vi "EditContact.vi"(7 "LabVIEW Web Service Request":refnum<class "Web Request.lvclass">) -> ()   [LabVIEW 2014]
doc: "This HTTP Method VI accepts a contact as form post data and either updates an existing contact or inserts a new one into the address book data store. It then redirects back to the contact list."
uses:
  <vilib>/wsapi/Web Request.lvclass
  DataManager/StateStore/Controls/DataFunction.ctl
panel:
  # "Because this is an HTTP Method VI, LabVIEW Web Service Request is populated automatically."
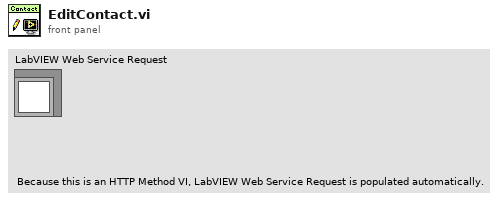
[diagram p1: front panel]
types:
  T1 = typedef "DataFunction.ctl" = enum16{"Initialise", "Release", "Get Data", "Set Data", "Preview Data"}
  T2 = typedef "CData Core Control.ctl" = cluster{"train_data_array":cluster{"uuid":string, "int":i32, "posit_array":cluster{"x":dbl, "y":dbl, "z":dbl}[]}[], "train_control_array":cluster{"uuid":string, "throttle":dbl, "brake":dbl, "horn":dbl, "wait":dbl, "name":string, "mode":string, "dest":string}[], "switch_data_array":cluster{"switch_posit":cluster{"x":dbl, "y":dbl, "z":dbl}, "manual":bool}[], "switch_control_array":cluster{"switch_posit":cluster{"x":dbl, "y":dbl, "z":dbl}, "switch":bool, "invert":bool, "wait":dbl}[]}
  T3 = cluster{"train_data":cluster{"uuid":string, "int":i32, "posit_array":cluster{"x":dbl, "y":dbl, "z":dbl}[]}, "train_control":cluster{"uuid":string, "throttle":dbl, "brake":dbl, "horn":dbl, "wait":dbl, "name":string, "mode":string, "dest":string}}
  T4 = typedef "Contact Data.lvlib/DestinationCluster.ctl" = cluster{"Desination":string, "DestControls":T5, "Timer":u32, "Set Timer":u32, "Time Stamp":timestamp, "Repeat?":bool, "Optional Data":string, "Distance":dbl}
  T5 = typedef "Contact Data.lvlib/DesinationControls.ctl" = enum16{"Tracker", "Manual", "Stop", "Station DateTime", "Station Timer", "Maintain"}
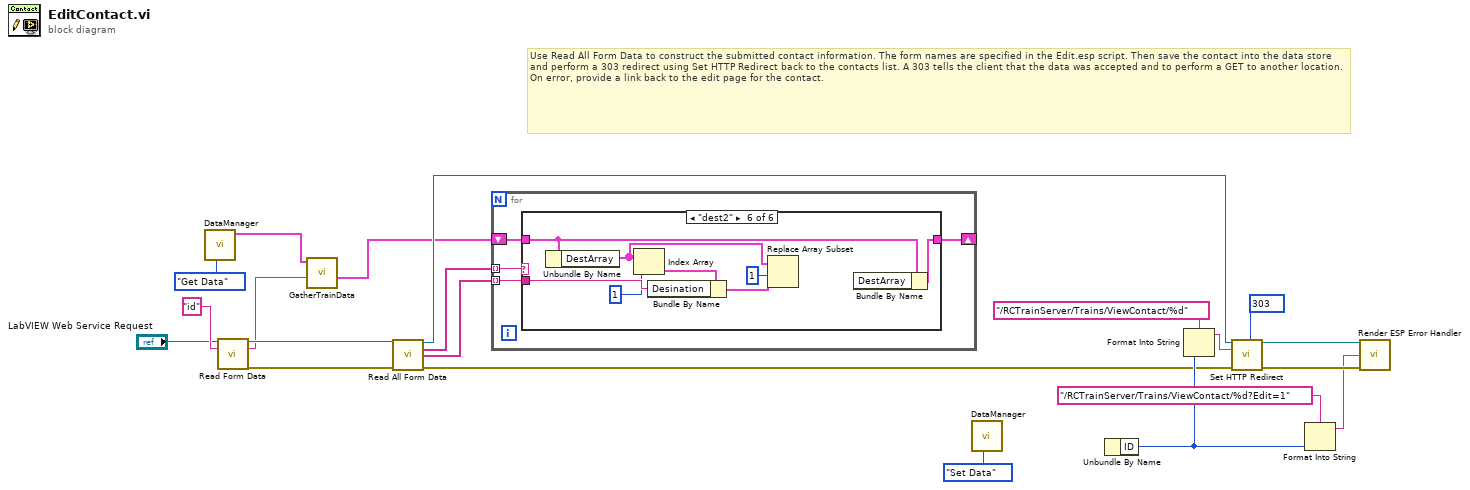
[diagram p0: block diagram]
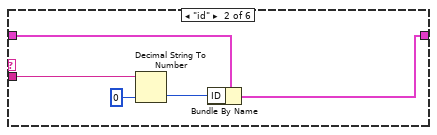
[diagram p3: hidden frame]
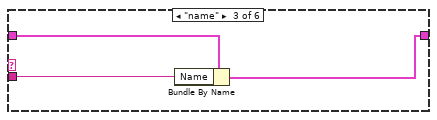
[diagram p4: hidden frame]
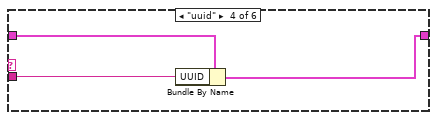
[diagram p5: hidden frame]
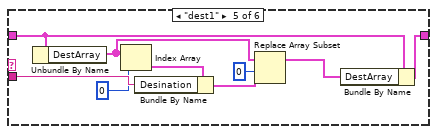
[diagram p6: hidden frame]
diagram:
  w21 = 303 items=["100"=100, "101"=101, "200"=200, "201"=201, "202"=202, "203"=203, "204"=204, "205"=205, "206"=206, "300"=300, "301"=301, "302"=302, "303"=303, "304"=304, "305"=305, "306"=306, "307"=307, "400"=400, "401"=401, "402"=402, "403"=403, "404"=404, "405"=405, "406"=406, "407"=407, "408"=408, "409"=409, "410"=410, "411"=411, "412"=412, "413"=413, "414"=414, "415"=415, "416"=416, "417"=417, "500"=500, "501"=501, "502"=502, "503"=503, "504"=504, "505"=505] ("response code (307)")
  # "Use Read All Form Data to construct the submitted contact information. The form names are specified in the Edit.esp script. Then save the contact into the data store and perform a 303 redirect using Set HTTP Redirect back to the contacts list. A 303 tells the client that the data was accepted and to perform a GET to another location. On error, provide a link back to the edit page for the contact."
  n1 = call "DataManager.vi"("DataFunction"=DataFunction."Get Data") -> ("CData Out"=w5:T2)  [unwired: 9 in, 1 out]
  n2 = call <vilib>:"Read Form Data.vi"("LabVIEW Web Service Request"="LabVIEW Web Service Request", "key"="id") -> ("LabVIEW Web Service Request out"=w11:refnum<class "Web Request.lvclass">, "value"=w6:string, "error out"=w10:errorcluster)  [unwired: 10 in, 1 out]
  n3 = call "GatherTrainData.vi"("uuid"=w6, "CData Out"=w5) -> ("Cluster"=w3:T3)  [unwired: 7 in, 2 out]
  n4 = call <vilib>:"Read All Form Data.vi"("LabVIEW Web Service Request"=w11, "error in (no error)"=w10) -> ("LabVIEW Web Service Request out"=w17:refnum<class "Web Request.lvclass">, "Key"=w19:string[], "Value"=w18:string[], "error out"=w1:errorcluster)  [unwired: 9 in, 1 out]
  n5 = for {
    tunnel: w19 -> [w25] mode=indexing
    tunnel: w18 -> [w24] mode=indexing
    shift-right: [w22] -> _
    shift-left: w3 -> [w23]
    n6 = case shown="\"dest2\"" w25 {
      tunnel: w24 -> [_ w29 w32 w36 w43 w51]
      tunnel: w23 -> [w26 w31 w34 w37 w45 w53]
      tunnel: [w26 w30 w33 w35 w46 w54] -> w22
      frame Default {
      }
      frame "id" {
        n7 = Decimal String To Number(string=w29, default (0L)=u32 0 ("default (0 I32)")) -> (number=w28:u32)  [unwired: 1 in, 1 out]
        n8 = Bundle By Name(cluster=w31, "ID"=w28) -> (w30:T3)
      }
      frame "name" {
        n9 = Bundle By Name(cluster=w34, "Name"=w32) -> (w33:T3)
      }
      frame "uuid" {
        n10 = Bundle By Name(cluster=w37, "UUID"=w36) -> (w35:T3)
      }
      frame "dest1" {
        n11 = Unbundle By Name(w45) -> ("DestArray"=w41:T4[])
        n12 = Index Array(array=w41, index=0) -> (element=w44:T4)
        n13 = Bundle By Name(cluster=w44, "Desination"=w43) -> (w39:T4)
        n14 = Replace Array Subset(array=w41, new element=w39, index=0) -> (w38:T4[])
        n15 = Bundle By Name(cluster=w45, "DestArray"=w38) -> (w46:T3)
      }
      frame "dest2" {
        n16 = Unbundle By Name(w53) -> ("DestArray"=w49:T4[])
        n17 = Index Array(array=w49, index=1) -> (element=w52:T4)
        n18 = Bundle By Name(cluster=w52, "Desination"=w51) -> (w47:T4)
        n19 = Replace Array Subset(array=w49, new element=w47, index=1) -> ()  [unwired: 1 out]
        n20 = Bundle By Name(cluster=w53) -> (w54:T3)  [unwired: 1 in]
      }
    }
  }
  n21 = call "DataManager.vi"("DataFunction"=DataFunction."Set Data") -> ()  [unwired: 9 in, 2 out]
  n22 = Unbundle By Name() -> ("ID"=w9:u32)  [unwired: 1 in]
  n23 = Format Into String(format string="/RCTrainServer/Trains/ViewContact/%d" ("redirect URL"), w9) -> (resulting string=w7:string)  [unwired: 2 in, 1 out]
  n24 = call <vilib>:"Set HTTP Redirect.vi"("LabVIEW Web Service Request"=w17, "redirect URL"=w7, "response code (307)"=w21, "error in (no error)"=w1) -> ("LabVIEW Web Service Request out"=w16:refnum<class "Web Request.lvclass">, "error out"=w15:errorcluster)  [unwired: 10 in]
  n25 = Format Into String(format string="/RCTrainServer/Trains/ViewContact/%d?Edit=1" ("Link"), w9) -> (resulting string=w14:string)  [unwired: 2 in, 1 out]
  n26 = call "Render ESP Error Handler.vi"("LabVIEW Web Service Request"=w16, "Link"=w14, "error in (no error)"=w15) -> ()  [unwired: 11 in, 2 out]
